vi "MVE Add or Overwrite Variable.vi"(5 "Array":refnum<vi>[](array[refnum]), 7 "Array 2":string[](array[string]), 8 "error IO":errorcluster, 10 "Name":string, 11 "ProjectItem Refnum":refnum<vi>) -> (0 "error out":errorcluster, 3 "AddItem":refnum<vi>)   [LabVIEW 2016]
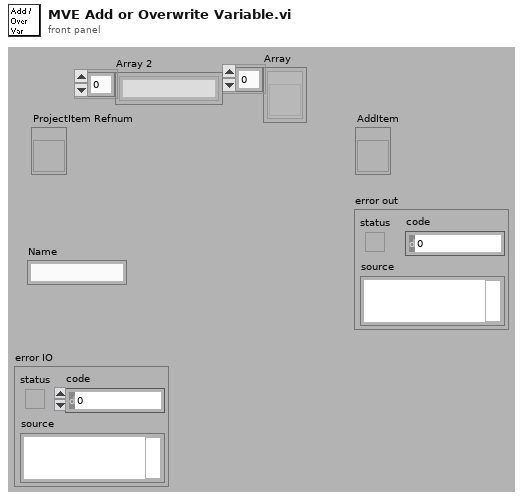
[diagram p1: front panel]
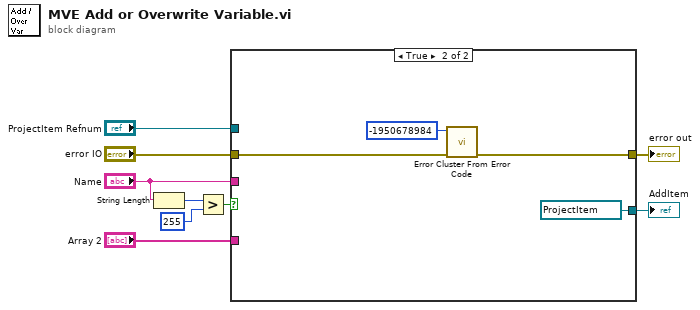
[diagram p0: block diagram]
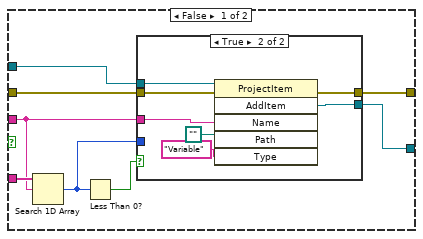
[diagram p2: hidden frame]
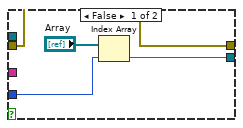
[diagram p3: hidden frame]
diagram:
  n1 = String Length(string="Name") -> (length=w4:i32)
  n2 = Greater?(x=w4, y=255) -> (0:w1:bool)
  n3 = case shown="True" w1 {
    tunnel: [w17 refnum<vi> refnum ("AddItem")] -> w9
    tunnel: [w16 w30] -> w8
    tunnel: "error IO" -> [w15 w32]
    tunnel: "Array 2" -> [w14 _]
    tunnel: "Name" -> [w13 _]
    tunnel: "ProjectItem Refnum" -> [w10 _]
    frame False {
      n4 = Search 1D Array(1D array=w14, element=w13) -> (index of element=w11:i32)  [unwired: 1 in]
      n5 = Less Than 0?(x=w11) -> (x < 0?=w12:bool)
      n6 = case shown="True" w12 {
        tunnel: w15 -> [w18 w28]
        tunnel: [w18 w27] -> w16
        tunnel: w13 -> [_ w24]
        tunnel: [w19 w23] -> w17
        tunnel: w10 -> [_ w22]
        tunnel: w11 -> [w20 _]
        frame False {
          n7 = Index Array(array="Array", index=w20) -> (element=w19:refnum<vi>)
        }
        frame True {
          n8 = invoke class="ProjectItem" method="AddItem"(reference=w22, error in=w28, "Name"=w24, "Path"=path "", "Type"="Variable") -> (error out=w27:errorcluster, "AddItem"=w23:refnum<vi>)  [unwired: 1 in, 4 out]
        }
      }
    }
    frame True {
      n9 = call <vilib>:"Error Cluster From Error Code.vi"("error in (no error)"=w32, "error code (0)"=-1950678984) -> ("error out"=w30:errorcluster)  [unwired: 7 in]
    }
  }
  "AddItem" <- w9
  "error out" <- w8
